vi "Set axis.vi"(6 "Accuracy (mm)":dbl=0.00023, 8 "error in":errorcluster, 9 "Axis to move":string(combo)="X", 10 "New axis pos (mm)":dbl, 11 "Stage VISA in":refnum<visa-resource-name>) -> (0 "error out":errorcluster, 3 "Stage VISA out":refnum<visa-resource-name>)   [LabVIEW 2017]
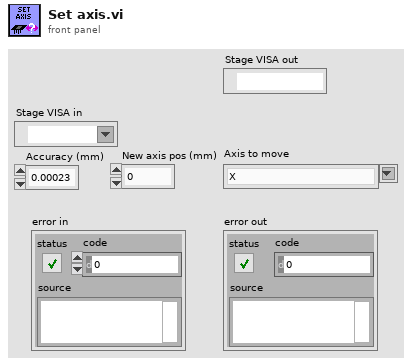
[diagram p1: front panel]
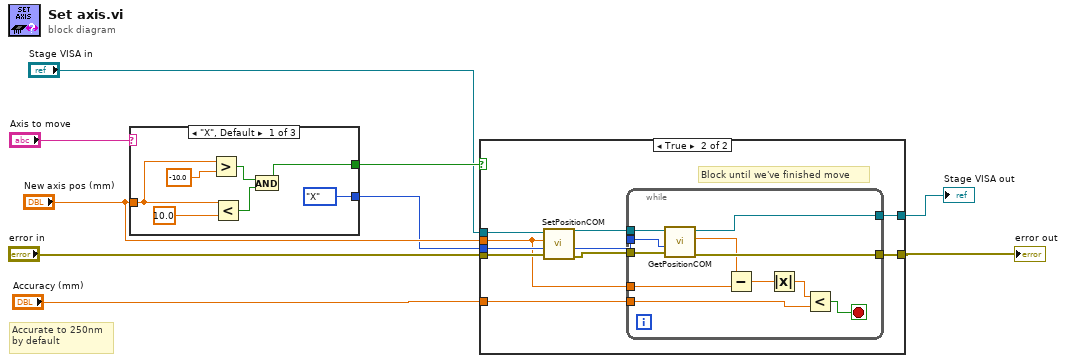
[diagram p0: block diagram]
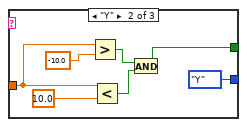
[diagram p3: hidden frame]
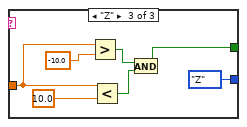
[diagram p4: hidden frame]
diagram:
  # "Accurate to 250nm\nby default"
  n1 = case shown="\"X\", Default" "Axis to move" {
    tunnel: "New axis pos (mm)" -> [w12 w19 w26]
    tunnel: [w13 w20 w27] -> w7
    tunnel: [enum16{"X", "Y", "Z"}."X" ("Axis") enum16{"X", "Y", "Z"}."Y" ("Axis") enum16{"X", "Y", "Z"}."Z" ("Axis")] -> w5
    frame "X", Default {
      n2 = Greater?(x=w12, y=-10.0) -> (0:w15:bool)
      n3 = Less?(x=w12, y=10.0 ("x")) -> (x < y?=w14:bool)
      n4 = And(x=w15, y=w14) -> (x .and. y?=w13:bool)
    }
    frame "Y" {
      n5 = Greater?(x=w19, y=-10.0) -> (0:w22:bool)
      n6 = Less?(x=w19, y=10.0 ("x")) -> (x < y?=w21:bool)
      n7 = And(x=w22, y=w21) -> (x .and. y?=w20:bool)
    }
    frame "Z" {
      n8 = Greater?(x=w26, y=-10.0) -> (0:w29:bool)
      n9 = Less?(x=w26, y=10.0 ("x")) -> (x < y?=w28:bool)
      n10 = And(x=w29, y=w28) -> (x .and. y?=w27:bool)
    }
  }
  n11 = case shown="True" w7 {
    tunnel: "error in" -> [w32 w41]
    tunnel: [w32 w39] -> w4
    tunnel: "New axis pos (mm)" -> [_ w33]
    tunnel: w5 -> [_ w38]
    tunnel: "Stage VISA in" -> [w31 w36]
    tunnel: [w31 w35] -> w2
    tunnel: "Accuracy (mm)" -> [_ w34]
    frame False {
      # "Don't move if we're outside +/- 10mm"
    }
    frame True {
      # "Block until we've finished move"
      n12 = call "SetPositionCOM.vi"("error in"=w41, "Axis"=w38, "Position (mm)"=w33, "VISA resource name"=w36) -> ("error out"=w40:errorcluster, "VISA resource name out"=w37:refnum<visa-resource-name>)  [unwired: 6 in]
      n13 = while {
        tunnel: w40 -> [w52]
        tunnel: [w51] -> w39
        tunnel: w38 -> [w50]
        tunnel: w37 -> [w49]
        tunnel: [w48] -> w35
        tunnel: w34 -> [w44]
        tunnel: w33 -> [w43]
        stop <- w45 stop-if-true
        n14 = call "GetPositionCOM.vi"("error in"=w52, "Axis"=w50, "VISA resource name"=w49) -> ("error out"=w51:errorcluster, "Position (mm)"=w42:dbl, "VISA resource name out"=w48:refnum<visa-resource-name>)  [unwired: 6 in]
        n15 = Subtract(x=w42, y=w43) -> (x-y=w47:dbl)
        n16 = Absolute Value(x=w47) -> (abs(x)=w46:dbl)
        n17 = Less?(x=w46, y=w44) -> (x < y?=w45:bool)
      }
    }
  }
  "error out" <- w4
  "Stage VISA out" <- w2
